vi "BLF_Time2Second.vi"(11 "Time":timestamp) -> (3 "Second":dbl)   [LabVIEW 2015]
uses:
  <vilib>/regexp/Match Regular Expression.xnode
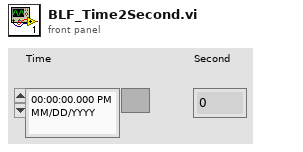
[diagram p1: front panel]
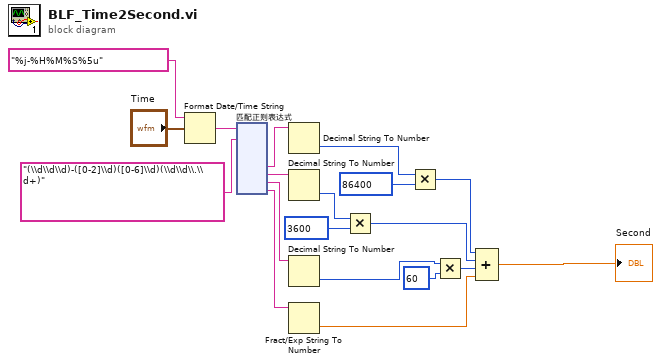
[diagram p0: block diagram]
diagram:
  n1 = Format Date/Time String(time format string (%c)="%j-%H%M%S%5u" ("时间格式字符串(%c)"), seconds (now)="Time") -> (date/time string=w2:string)  [unwired: 1 in]
  n2 = xnode "匹配正则表达式"("输入字符串"=w2, "正则表达式"="(\\d\\d\\d)-([0-2]\\d)([0-6]\\d)(\\d\\d\\.\\d+)") -> ("子匹配 1"=w3:string, "子匹配 2"=w4:string, "子匹配 3"=w5:string, "子匹配 4"=w6:string)  [unwired: 4 in, 5 out]
  n3 = Decimal String To Number(string=w3) -> (number=w15:i32)  [unwired: 2 in, 1 out]
  n4 = Decimal String To Number(string=w4) -> (number=w16:i32)  [unwired: 2 in, 1 out]
  n5 = Decimal String To Number(string=w5) -> (number=w1:i32)  [unwired: 2 in, 1 out]
  n6 = Fract/Exp String To Number(string=w6) -> (number=w17:dbl)  [unwired: 3 in, 1 out]
  n7 = Multiply(x=w16, y=3600) -> (x*y=w13:i32)
  n8 = Multiply(x=w15, y=86400) -> (x*y=w12:i32)
  n9 = Multiply(x=w1, y=60) -> (x*y=w14:i32)
  n10 = Compound Arithmetic op=ADD(w12, w13, w14, w17) -> (→"Second":dbl)
